vi "Convert String Value to Boolean.vi"(11 "Cell String":string(combo)) -> (3 "Boolean":bool)   [LabVIEW 2021]
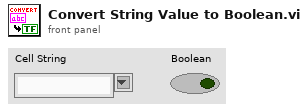
[diagram p1: front panel]
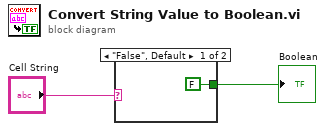
[diagram p0: block diagram]
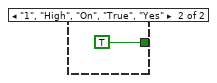
[diagram p2: hidden frame]
diagram:
  n1 = case shown="\"False\", Default" "Cell String" {
    tunnel: [FALSE TRUE] -> w2
    frame "False", Default {
    }
    frame "1", "High", "On", "True", "Yes" {
    }
  }
  "Boolean" <- w2
